vi "ChooseReceptorPass.vi"(6 "atacando ao contrário?":bool=TRUE, 8 "Impulso 2nd\nStriker Ativo":bool=TRUE, 10 "IA State Input":T2={"our_robots"=[], "enemy_robots"=[], "balls"=[], "geometry"={"line_width"=0, "field_length"=0, "field_width"=0, "boundary_width"=0, "referee_width"=0, "goal_width"=0, "goal_depth"=0, "goal_wall_width"=0, "center_circle_radius"=0, "defense_radius"=0, "defense_stretch"=0, "free_kick_from_defense_dist"=0, "penalty_spot_from_field_line_dist"=0, "penalty_line_from_spot_dist"=0}, "IA Judge"={"stage"="", "command"="", "our_goalie_id"=0.0, "enemy_goalie_id"=0.0, "command enum"=enum."Halt", "Time"=enum."Azul"}, "Received Timestamp"=timestamp(0 s since 1904-01-01), "Events"={"Touch"=FALSE, "Ball out"=FALSE, "id touch"=0.0, "Ball out of \nVision"=FALSE, "Ball inside \nGoalie area"=FALSE, "Robot not responding"=FALSE, "Robots responding status"=[1.0, 1.0, 1.0, 1.0, 1.0, 1.0], "Enemy Ball \nPossession"=FALSE, "Pass State"=FALSE, "id end of pass"=0.0, "Kick"=FALSE, "Id ini Possession"=0.0, "Ball Possesion"=FALSE, "Id Possesion"=0.0, "Direct Kick"=FALSE, "2nd Strk Ativo"=FALSE}}, 11 "AI Parameters":T1={"GotoKick"={"Dist do cone a frente"=150.0, "attacker farback"=1500.0, "Perto"=300.0, "min dist to kick"=150.0, "kick eps"=0.0, "Time to transition"=0.05}, "Attacker"={"CC chute"=0.09, "CC passe"=0.045, "Kick Force"=100.0, "ball-robot Kick"=200.0, "ball-robot Pass"=0.3, "drible\nAttk"=FALSE}, "Defender"={"D max"=1700.0, "Vel p/ robô av"=1000.0, "Kick Force"=100.0, "D atk-def"=0.0, "D farback"=0.0, "drible\ndef"=FALSE, "drible\ngoalie"=FALSE}, "Timeout"={"Field/v in x"=6.0, "Dist Robots"=300, "Dist up in y"=300}, "Pose Striker"={"dist"=200.0, "Numeric"=-4.0, "dist 2"=200.0, "drible\nstriker"=FALSE}, "Dist Stop"=300.0, "D ball out"=200, "D central gap "=150.0, "T pass"=0.0, "Force ++"=0.0, "range kick"=0.0, "Chute alto"=TRUE, "Marcador novo"=TRUE, "drible"=FALSE, "D drible"=300.0, "Versão Striker"=enum."3", "Defesa"=enum."ManMark", "Marcador"=enum."Marcar Segundo mais perigoso", "Receptor passe"=enum."2nd Striker", "Área"=enum."Quadrada", "Decisão\nsimples?"=FALSE} {"D drible" format="%#_13g"; "D central gap" format="%#_13g"; "Dist Stop" format="%#_13g"; "Pose Striker"."Numeric" format="%#_13g"; "Defender"."Kick Force" format="%#_13g"; "Defender"."Vel p/ robô av" format="%#_13g"; "Attacker"."ball-robot Kick" format="%#_13g"; "Attacker"."Kick Force" format="%#_13g"; "Attacker"."CC passe" format="%#_13g"; "Attacker"."CC chute" format="%#_13g"; "GotoKick"."kick eps" format="%#_13g"; "GotoKick"."min dist to kick" format="%#_13g"; "GotoKick"."Perto" format="%#_13g"; "GotoKick"."attacker farback" format="%#_13g"; "GotoKick"."Dist do cone a frente" format="%#_13g"}) -> (3 "Receptor passe":enum16{"Auto", "2nd Striker", "Striker"}(ring)=enum."Striker")   [LabVIEW 2017]
uses:
  Core/AI Input.ctl
  Core/AI Robot.ctl
  Functions Enum.ctl
  AttackerStates.ctl
  Path Planning/RRT/PathDests.ctl
  Path Planning/RRT/PathDest.ctl
  Core/AI Ball.ctl
  Core/Field Size.ctl
  Core/AI Judge.ctl
  Command Enum.ctl
  Util/Events/Events.ctl
  AI Parameters.ctl
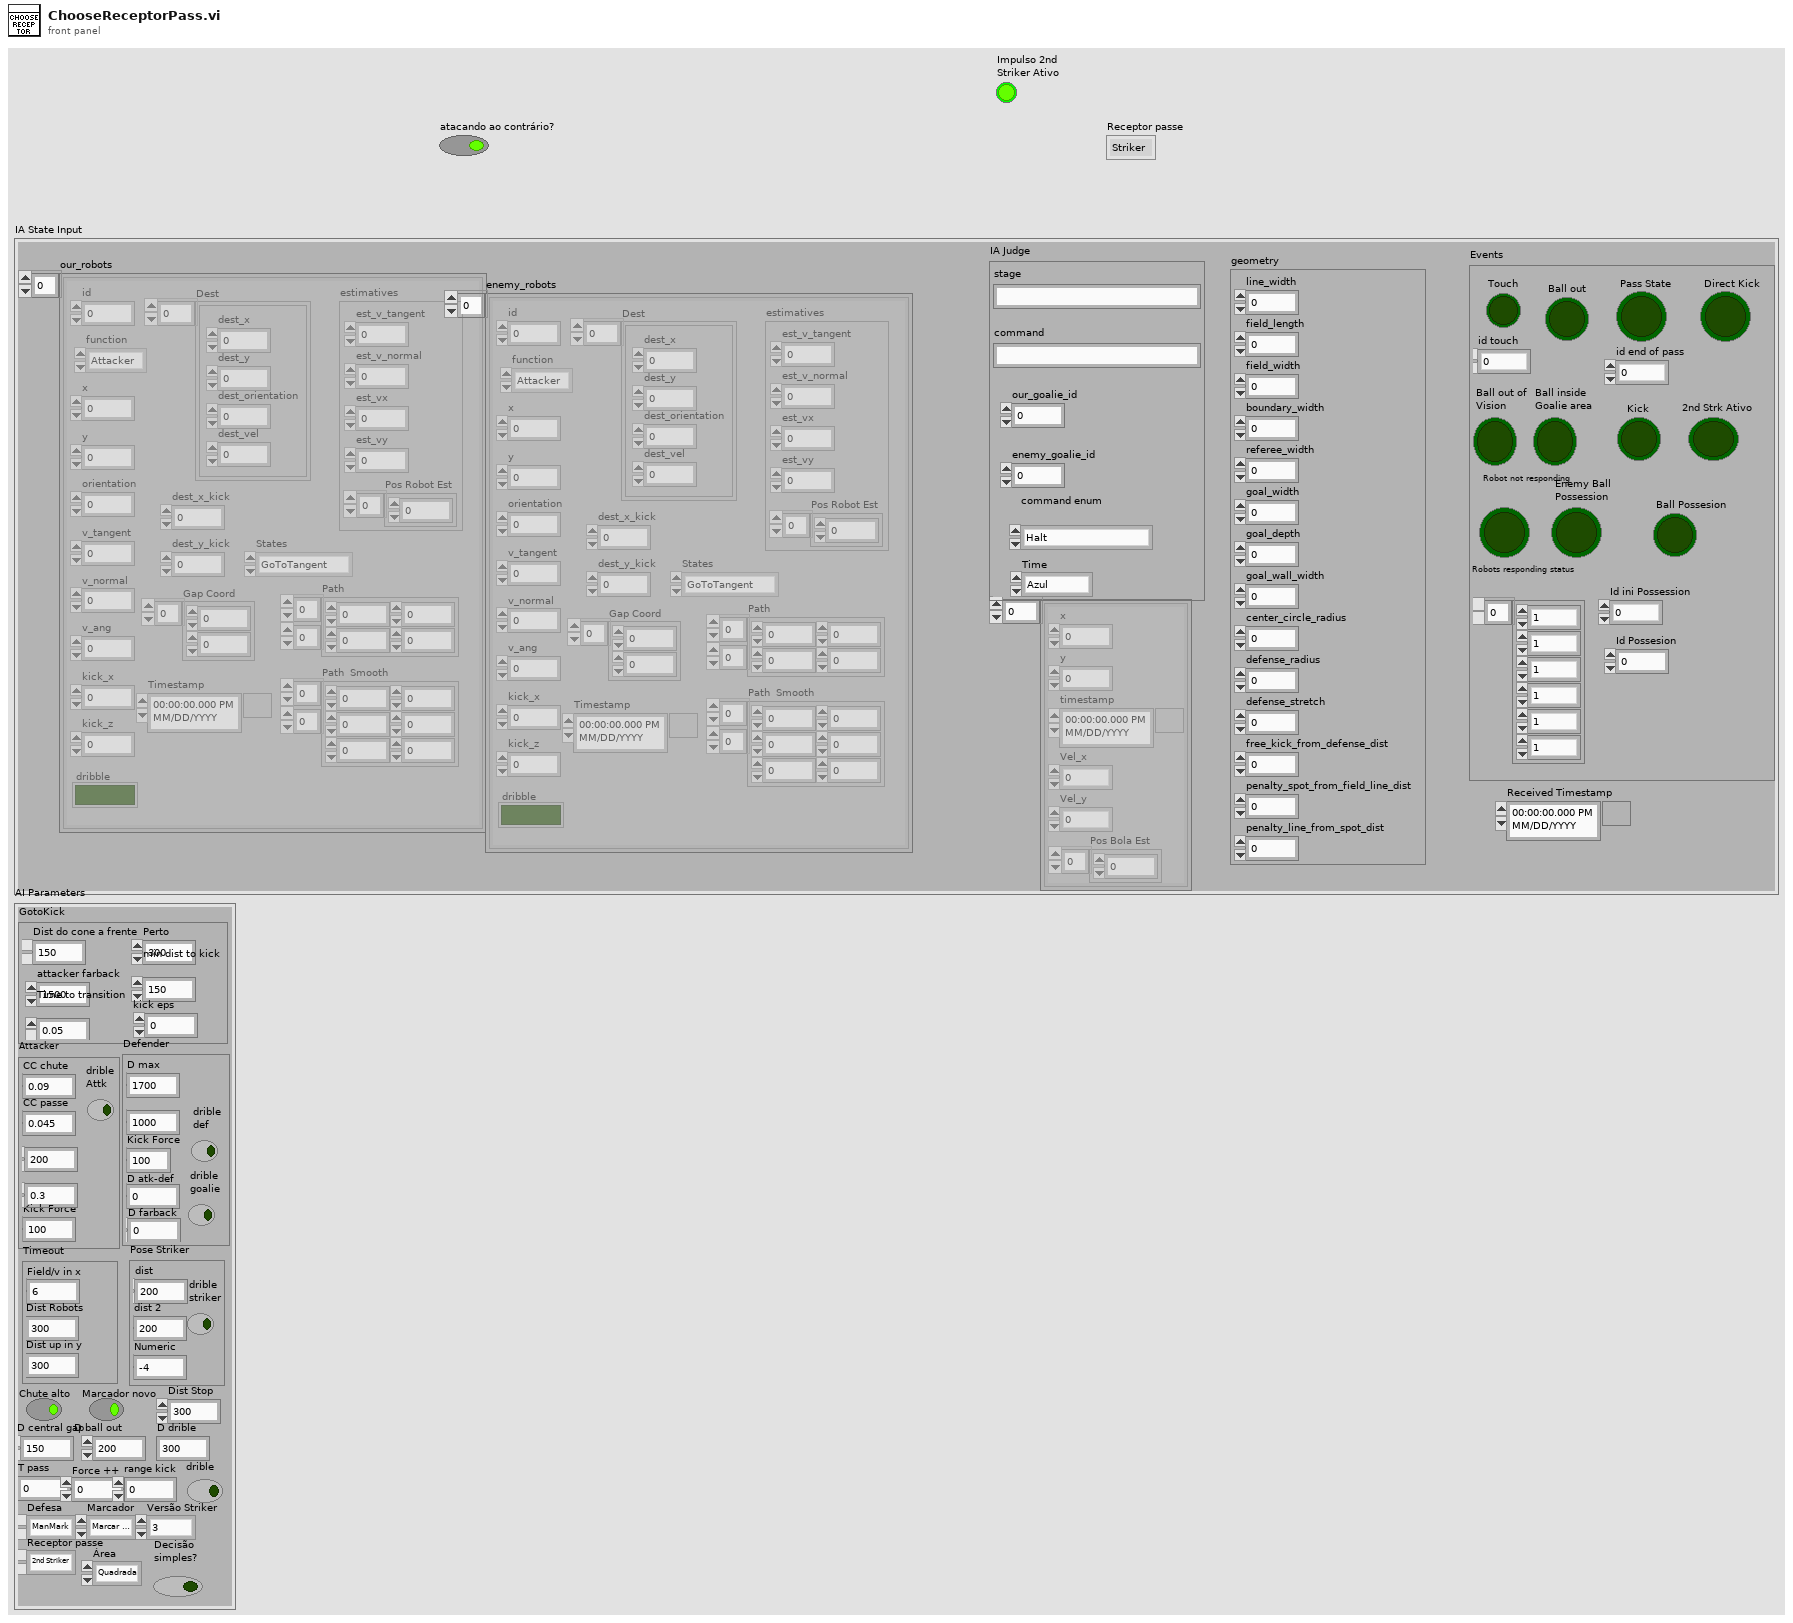
[diagram p1: front panel]
types:
  T1 = typedef "AI Parameters.ctl" = cluster{"GotoKick":cluster{"Dist do cone a frente":dbl, "attacker farback":dbl, "Perto":dbl, "min dist to kick":dbl, "kick eps":dbl, "Time to transition":dbl}, "Attacker":cluster{"CC chute":dbl, "CC passe":dbl, "Kick Force":dbl, "ball-robot Kick":dbl, "ball-robot Pass":dbl, "drible\nAttk":bool}, "Defender":cluster{"D max":dbl, "Vel p/ robô av":dbl, "Kick Force":dbl, "D atk-def":dbl, "D farback":dbl, "drible\ndef":bool, "drible\ngoalie":bool}, "Timeout":cluster{"Field/v in x":dbl, "Dist Robots":u32, "Dist up in y":u32}, "Pose Striker":cluster{"dist":dbl, "Numeric":dbl, "dist 2":dbl, "drible\nstriker":bool}, "Dist Stop":dbl, "D ball out":i32, "D central gap ":dbl, "T pass":dbl, "Force ++":dbl, "range kick":dbl, "Chute alto":bool, "Marcador novo":bool, "drible":bool, "D drible":dbl, "Versão Striker":enum16{"Auto", "3", "2", "1"}, "Defesa":enum16{"ManMark", "Barreira"}, "Marcador":enum16{"Marcar Segundo mais perigoso", "Marcar o mais perigoso"}, "Receptor passe":enum16{"Auto", "2nd Striker", "Striker"}, "Área":enum16{"Quadrada", "Circular"}, "Decisão\nsimples?":bool}
  T2 = typedef "AI Input.ctl" = cluster{"our_robots":T3[], "enemy_robots":T3[], "balls":T8[], "geometry":T9, "IA Judge":T10, "Received Timestamp":timestamp, "Events":T12}
  T3 = typedef "AI Robot.ctl" = cluster{"id":u32, "function":T4, "x":dbl, "y":dbl, "orientation":dbl, "v_tangent":dbl, "v_normal":dbl, "v_ang":dbl, "kick_x":dbl, "kick_z":dbl, "dribble":bool, "Timestamp":timestamp, "estimatives":cluster{"est_v_tangent":dbl, "est_v_normal":dbl, "est_vx":dbl, "est_vy":dbl, "Pos Robot Est":dbl[]}, "dest_x_kick":dbl, "dest_y_kick":dbl, "Gap Coord":dbl[], "States":T5, "Path ":dbl[][], "Path  Smooth":dbl[][], "Dest":T6}
  T4 = typedef "Functions Enum.ctl" = enum16{"2nd Striker", "Attacker", "Goalie", "Defender", "Striker", "Goto 0", "Dummy", "Kicker", "ZigZag 0", "ZigZag 1", "ZigZag 2", "ZigZag 3", "ZigZag 4", "ZigZag 5", "ZigZag 6", "ZigZag 7", "ZigZag 8", ""}
  T5 = typedef "AttackerStates.ctl" = enum16{"Pass", "GoToTangent", "BallGetting", "GoToKick", ""}
  T6 = typedef "PathDests.ctl" = T7[]
  T7 = typedef "PathDest.ctl" = cluster{"dest_x":dbl, "dest_y":dbl, "dest_orientation":dbl, "dest_vel":dbl}
  T8 = typedef "AI Ball.ctl" = cluster{"x":dbl, "y":dbl, "timestamp":timestamp, "Vel_x":dbl, "Vel_y":dbl, "Pos Bola Est":dbl[]}
  T9 = typedef "Field Size.ctl" = cluster{"line_width":u32, "field_length":u32, "field_width":u32, "boundary_width":u32, "referee_width":u32, "goal_width":u32, "goal_depth":u32, "goal_wall_width":u32, "center_circle_radius":u32, "defense_radius":u32, "defense_stretch":u32, "free_kick_from_defense_dist":u32, "penalty_spot_from_field_line_dist":u32, "penalty_line_from_spot_dist":u32}
  T10 = typedef "AI Judge.ctl" = cluster{"stage":string, "command":string, "our_goalie_id":dbl, "enemy_goalie_id":dbl, "command enum":T11, "Time":enum16{"Azul", "Amarelo"}}
  T11 = typedef "Command Enum.ctl" = enum16{"Halt", "Stop", "Force Start", "PKA Normal Start", "Prepare Kickoff Ally", "PKE Normal Start", "Prepare Kickoff Enemy", "Prepare Penalty Ally", "PPA Normal Start", "Prepare Penalty Enemy", "PPE Normal Start", "Direct Free Enemy", "Direct Free Ally", "Indirect Free Enemy", "Indirect Free Ally", "Timeout Enemy", "Timeout Ally", "Goal Enemy", "Goal Ally", "Ball Placement Enemy", "Ball Placement Ally", "Normal Half Time", "Extra Time Break", "Extra Half Time", "None", "Post Game"}
  T12 = typedef "Events.ctl" = cluster{"Touch":bool, "Ball out":bool, "id touch":dbl, "Ball out of \nVision":bool, "Ball inside \nGoalie area":bool, "Robot not responding":bool, "Robots responding status":dbl[], "Enemy Ball \nPossession":bool, "Pass State":bool, "id end of pass":dbl, "Kick":bool, "Id ini Possession":dbl, "Ball Possesion":bool, "Id Possesion":dbl, "Direct Kick":bool, "2nd Strk Ativo":bool}
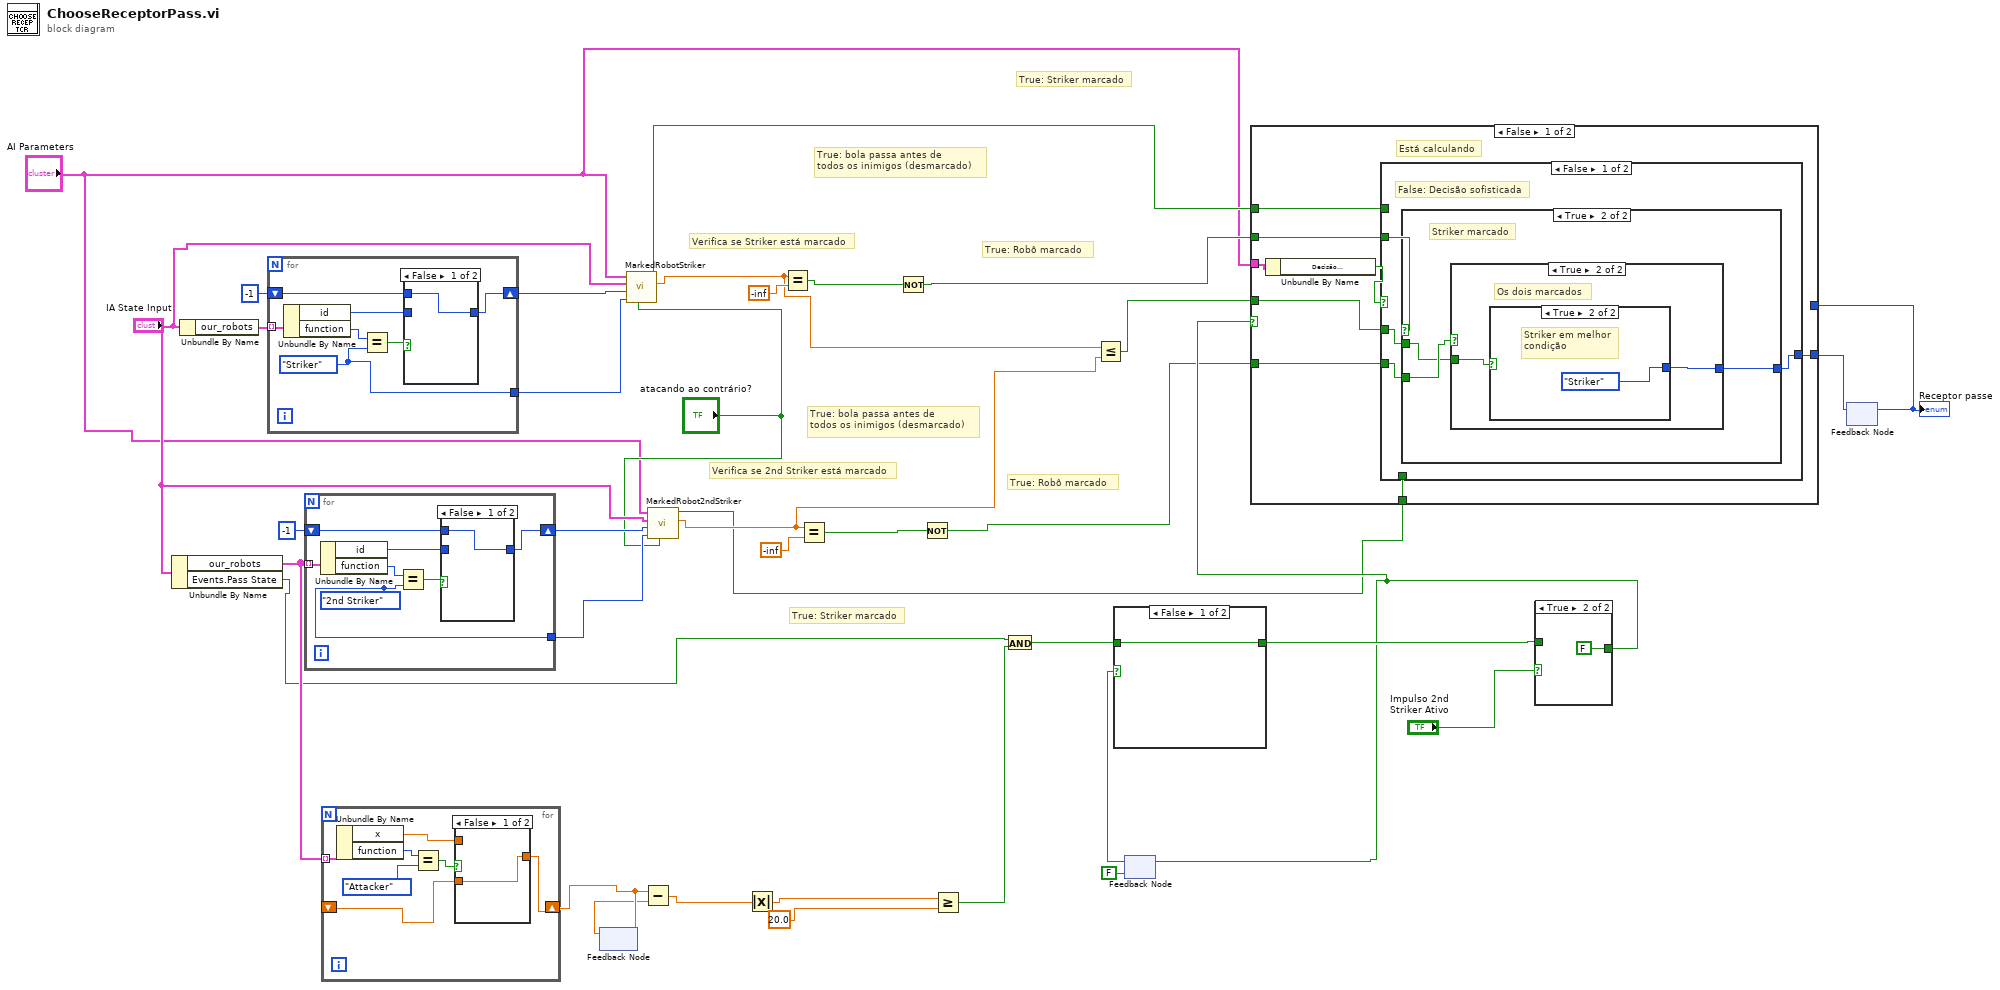
[diagram p0: block diagram]
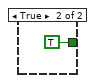
[diagram p3: hidden frame]
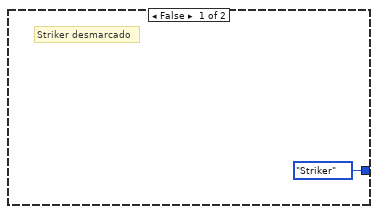
[diagram p5: hidden frame]
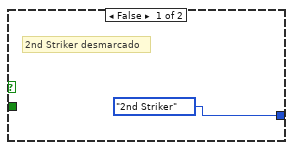
[diagram p6: hidden frame]
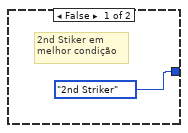
[diagram p7: hidden frame]
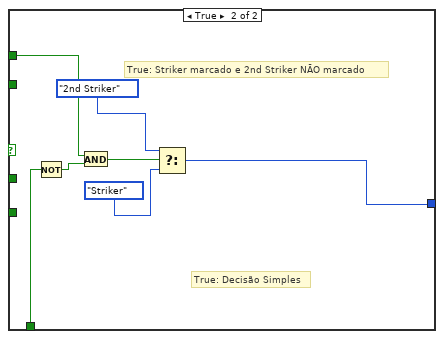
[diagram p8: hidden frame]
diagram:
  # "True: Striker marcado"
  # "True: Striker marcado"
  # "True: Robô marcado"
  # "True: bola passa antes de \ntodos os inimigos (desmarcado)"
  # "True: Robô marcado"
  # "True: bola passa antes de \ntodos os inimigos (desmarcado)"
  # "Verifica se 2nd Striker está marcado"
  # "Verifica se Striker está marcado"
  n1 = Unbundle By Name("IA State Input") -> ("our_robots"=w29:T3[], "Events.Pass State"=w20:bool)
  n2 = Unbundle By Name("IA State Input") -> ("our_robots"=w37:T3[])
  n3 = for {
    tunnel: w37 -> [w44] mode=indexing
    shift-right: [w41] -> w35
    shift-left: -1 ("id") -> [w39]
    tunnel: [w38] -> w16
    w38 = Functions_Enum."Striker" ("y")
    n4 = Unbundle By Name(w44) -> ("id"=w40:u32, "function"=w43:T4)
    n5 = Equal?(x=w43, y=w38) -> (x = y?=w42:bool)
    n6 = case shown="False" w42 {
      tunnel: [w45 w46] -> w41
      tunnel: w40 -> [_ w46]
      tunnel: w39 -> [w45 _]
      frame False {
      }
      frame True {
      }
    }
  }
  n7 = for {
    tunnel: w29 -> [w53] mode=indexing
    shift-right: [w50] -> w33
    shift-left: -1 ("id") -> [w48]
    tunnel: [w47] -> w17
    w47 = Functions_Enum."2nd Striker" ("y")
    n8 = Unbundle By Name(w53) -> ("id"=w49:u32, "function"=w52:T4)
    n9 = Equal?(x=w52, y=w47) -> (x = y?=w51:bool)
    n10 = case shown="False" w51 {
      tunnel: [w54 w55] -> w50
      tunnel: w49 -> [_ w55]
      tunnel: w48 -> [w54 _]
      frame False {
      }
      frame True {
      }
    }
  }
  n11 = for {
    tunnel: w29 -> [w62] mode=indexing
    shift-right: [w58] -> w28
    shift-left: _ -> [w56]
    n12 = Unbundle By Name(w62) -> ("x"=w57:dbl, "function"=w61:T4)
    n13 = Equal?(x=w61, y=Functions_Enum."Attacker") -> (x = y?=w59:bool)
    n14 = case shown="False" w59 {
      tunnel: [w63 w64] -> w58
      tunnel: w57 -> [_ w64]
      tunnel: w56 -> [w63 _]
      frame False {
      }
      frame True {
      }
    }
  }
  n15 = feedback-in #1(w28) -> ()
  n16 = feedback #1() -> (w27:dbl)  [unwired: 1 in]
  n17 = call "MarkedRobotStriker.vi"("atacando ao contrário?"="atacando ao contrário?", "Função"=w16, "id"=w35, "IA State Input"="IA State Input", "AI Parameters"="AI Parameters") -> ("Dif. tempo\ninimigo bola"=w6:dbl, "Robô marcado?"=w3:bool)  [unwired: 4 in, 1 out]
  n18 = Subtract(x=w28, y=w27) -> (x-y=w26:dbl)
  n19 = call "MarkedRobot2ndStriker.vi"("atacando ao contrário?"="atacando ao contrário?", "Função"=w17, "id"=w33, "IA State Input"="IA State Input", "AI Parameters"="AI Parameters") -> ("Dif. tempo\ninimigo bola"=w5:dbl, "Robô marcado?"=w2:bool)  [unwired: 4 in, 1 out]
  n20 = Absolute Value(x=w26) -> (abs(x)=w25:dbl)
  n21 = Equal?(x=w6, y=-inf) -> (x = y?=w10:bool)
  n22 = Equal?(x=w5, y=-inf) -> (x = y?=w8:bool)
  n23 = Not(x=w10) -> (.not. x?=w9:bool)
  n24 = Not(x=w8) -> (.not. x?=w7:bool)
  n25 = Greater Or Equal?(x=w25, y=20.0) -> (x >= y?=w23:bool)
  n26 = And(x=w20, y=w23) -> (x .and. y?=w21:bool)
  n27 = Less Or Equal?(x=w6, y=w5) -> (x <= y?=w12:bool)
  n28 = feedback #2(FALSE) -> (w14:bool)
  n29 = case shown="False" w14 {
    tunnel: [w65 TRUE] -> w19
    tunnel: w21 -> [w65 _]
    frame False {
    }
    frame True {
    }
  }
  n30 = case shown="True" "Impulso 2nd\nStriker Ativo" {
    tunnel: [w67 FALSE] -> w18
    tunnel: w19 -> [w67 _]
    frame False {
    }
    frame True {
    }
  }
  n31 = feedback-in #2(w18) -> ()
  n32 = feedback #3() -> (w30:enum16{"Auto", "2nd Striker", "Striker"})  [unwired: 1 in]
  "Receptor passe" <- w30
  n33 = case shown="False" w18 {
    tunnel: [w76 w97] -> w31
    tunnel: w30 -> [_ w97]
    tunnel: w9 -> [w75 _]
    tunnel: w7 -> [w74 _]
    tunnel: w12 -> [w73 _]
    tunnel: w3 -> [w72 _]
    tunnel: w2 -> [w71 _]
    tunnel: "AI Parameters" -> [w70 _]
    frame False {
      # "Está calculando"
      n34 = Unbundle By Name(w70) -> ("Decisão\nsimples?"=w69:bool)
      n35 = case shown="False" w69 {
        tunnel: [w80 w91] -> w76
        tunnel: w75 -> [w79 _]
        tunnel: w74 -> [w78 _]
        tunnel: w73 -> [w77 _]
        tunnel: w72 -> [_ w90]
        tunnel: w71 -> [_ w95]
        frame False {
          # "False: Decisão sofisticada"
          n36 = case shown="True" w79 {
            tunnel: [enum16{"Auto", "2nd Striker", "Striker"}."Striker" ("Receptor passe") w84] -> w80
            tunnel: w78 -> [_ w83]
            tunnel: w77 -> [_ w82]
            frame False {
              # "Striker desmarcado"
            }
            frame True {
              # "Striker marcado"
              n37 = case shown="True" w83 {
                tunnel: [enum16{"Auto", "2nd Striker", "Striker"}."2nd Striker" ("Receptor passe") w86] -> w84
                tunnel: w82 -> [_ w87]
                frame False {
                  # "2nd Striker desmarcado"
                }
                frame True {
                  # "Os dois marcados"
                  n38 = case shown="True" w87 {
                    tunnel: [enum16{"Auto", "2nd Striker", "Striker"}."2nd Striker" ("Receptor passe") enum16{"Auto", "2nd Striker", "Striker"}."Striker" ("Receptor passe")] -> w86
                    frame False {
                      # "2nd Stiker em\nmelhor condição"
                    }
                    frame True {
                      # "Striker em melhor\ncondição"
                    }
                  }
                }
              }
            }
          }
        }
        frame True {
          # "True: Decisão Simples"
          # "True: Striker marcado e 2nd Striker NÃO marcado"
          n39 = Not(x=w95) -> (.not. x?=w94:bool)
          n40 = And(x=w90, y=w94) -> (x .and. y?=w96:bool)
          n41 = Select(t=enum16{"Auto", "2nd Striker", "Striker"}."2nd Striker" ("Receptor passe"), s=w96, f=enum16{"Auto", "2nd Striker", "Striker"}."Striker" ("Receptor passe")) -> (s? t:f=w91:enum16{"Auto", "2nd Striker", "Striker"})
        }
      }
    }
    frame True {
      # "Já parou de calcular"
    }
  }
  n42 = feedback-in #3(w31) -> ()
